vi "GET_Zone_number_(offline).vi"(0 "Animal coordinates cluster in":T2, 1 "Mouse drawing parameters":T3, 2 "Size of the image (480x480)":T4={"Numeric Control"=480.0, "Numeric Control"=480.0}, 3 "error in (no error)":T1, 4 "Array of the pixel to zone correspondences":T5) -> (5 "Animal coordinates cluster out":T2, 6 "error out":T1)   [LabVIEW 2018, in "Tracker.lvlib"]
uses:
  Tracker.lvlib
  Controls/CTL_Pixel_to_Zone_array.ctl
  Controls/CTL_Mouse_Draw_Params.ctl
  Controls/CTL_Animal_Coordinates_and_Speed_(arr).ctl
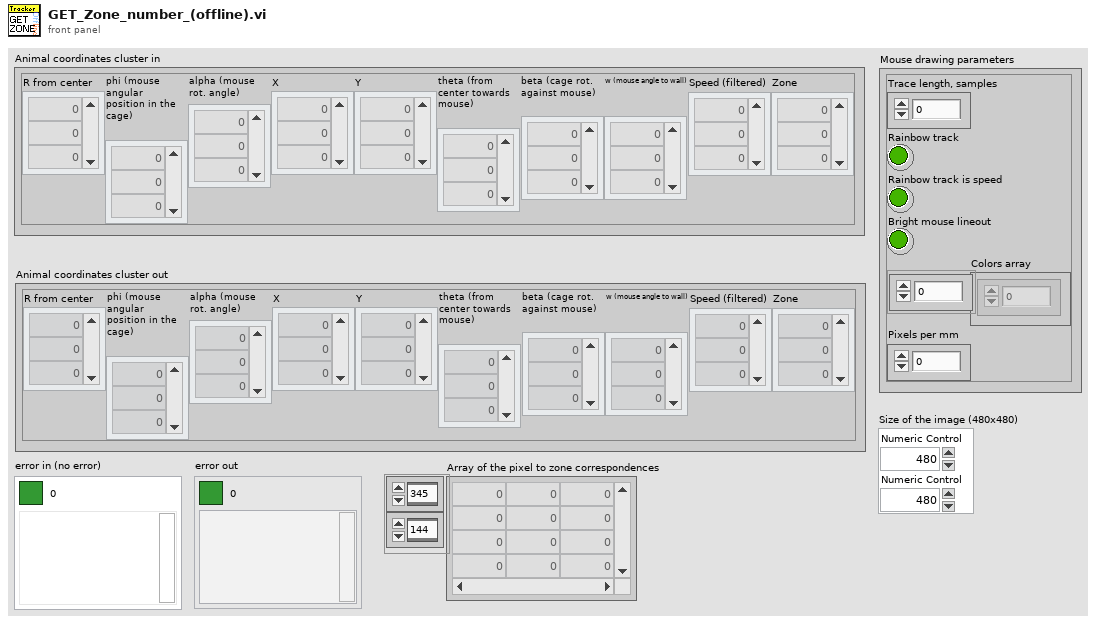
[diagram p1: front panel]
types:
  T1 = cluster{"Boolean Round":bool, "code":i32, "source":string}
  T2 = typedef "Tracker.lvlib/CTL_Animal_Coordinates_and_Speed_(arr).ctl" = cluster{"R from center":dbl[], "phi (mouse angular position in the cage)":dbl[], "alpha (mouse rot. angle)":dbl[], "X":dbl[], "Y":dbl[], "theta (from center towards mouse)":dbl[], "beta (cage rot. against mouse)":dbl[], "w (mouse angle to wall)":dbl[], "Speed (filtered)":dbl[], "Zone":i8[]}
  T3 = typedef "Tracker.lvlib/CTL_Mouse_Draw_Params.ctl" = cluster{"Trace length, samples":u16, "Rainbow track":bool, "Rainbow track is speed":bool, "Bright mouse lineout":bool, "Colors array":u32[], "Pixels per mm":dbl}
  T4 = cluster{"Numeric Control":dbl, "Numeric Control":dbl}
  T5 = typedef "Tracker.lvlib/CTL_Pixel_to_Zone_array.ctl" = i8[][]
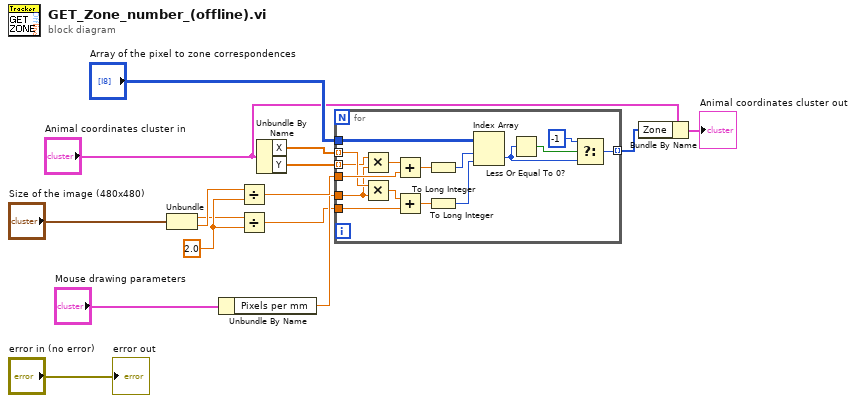
[diagram p0: block diagram]
diagram:
  w13 = 2.0
  n1 = Unbundle("Size of the image (480x480)") -> ("Numeric Control"=w4:dbl, "Numeric Control"=w14:dbl)
  n2 = Unbundle By Name("Mouse drawing parameters") -> ("Pixels per mm"=w5:dbl)
  n3 = Divide(x=w14, y=w13) -> (x/y=w12:dbl)
  n4 = Divide(x=w4, y=w13) -> (x/y=w3:dbl)
  n5 = Unbundle By Name("Animal coordinates cluster in") -> ("X"=w1:dbl[], "Y"=w2:dbl[])
  n6 = for {
    tunnel: w12 -> [w31]
    tunnel: "Array of the pixel to zone correspondences" -> [w27]
    tunnel: w1 -> [w23] mode=indexing
    tunnel: w2 -> [w22] mode=indexing
    tunnel: [w18] -> w9 mode=indexing
    tunnel: w5 -> [w17]
    tunnel: w3 -> [w16]
    n7 = Multiply(x=w22, y=w17) -> (x*y=w29:dbl)
    n8 = Multiply(x=w23, y=w17) -> (x*y=w30:dbl)
    n9 = Add(x=w29, y=w31) -> (x+y=w26:dbl)
    n10 = Add(x=w30, y=w16) -> (x+y=w28:dbl)
    n11 = To Long Integer(number=w26) -> (32bit integer=w24:i32)
    n12 = To Long Integer(number=w28) -> (32bit integer=w25:i32)
    n13 = Index Array(array=w27, index (row)=w24, index (col)=w25) -> (element=w20:i8)
    n14 = Less Or Equal To 0?(x=w20) -> (x <= 0?=w21:bool)
    n15 = Select(t=i8 -1, s=w21, f=w20) -> (s? t:f=w18:i8)
  }
  n16 = Bundle By Name(cluster="Animal coordinates cluster in", "Zone"=w9) -> (→"Animal coordinates cluster out":T2)
  "error out" <- "error in (no error)"
